vi "125_tcp_test.vi"() -> ()   [LabVIEW 2011]
panel:
  in  "CloseConnection?":bool
  out "length":i32
  out "error out":errorcluster
  out "data out":string
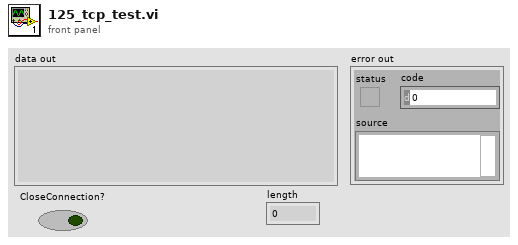
[diagram p1: front panel]
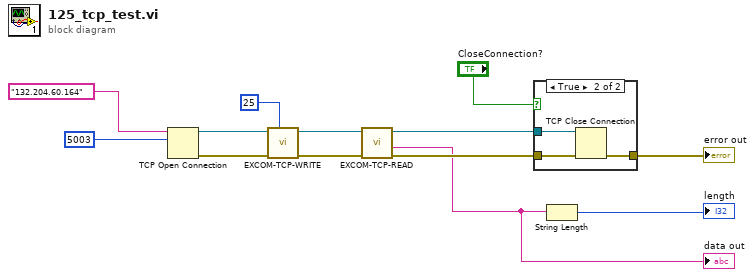
[diagram p0: block diagram]
diagram:
  n1 = TCP Open Connection(address="132.204.60.164", remote port or service name=u16 5003) -> (connection ID=w5:refnum<k5>, error out=w4:errorcluster)  [unwired: 3 in]
  n2 = call "EXCOM-TCP-WRITE.vi"("Commande #"=25, "Error IN"=w4, "connection ID"=w5) -> ("Error OUT"=w2:errorcluster, "connection ID out"=w3:refnum<k5>)  [unwired: 4 in, 2 out]
  n3 = call "EXCOM-TCP-READ.vi"("Error In"=w2, "connection ID"=w3) -> ("Error Out"=w9:errorcluster, "Response"=w7:string, "CID Out"=w8:refnum<k5>)  [unwired: 5 in]
  "data out" <- w7
  n4 = case shown="True" "CloseConnection?" {
    tunnel: [w14 w17] -> w11
    tunnel: w9 -> [w14 w16]
    tunnel: w8 -> [_ w15]
    frame False {
    }
    frame True {
      n5 = TCP Close Connection(connection ID=w15, error in (no error)=w16) -> (error out=w17:errorcluster)  [unwired: 1 in, 1 out]
    }
  }
  "error out" <- w11
  n6 = String Length(string=w7) -> (length=→"length":i32)
